vi "XCalib.vi"(7 "B [T]":dbl=1.0, 8 "error in (no error)":errorcluster, 10 "fileCalib":T1, 11 "DB calib":T10) -> (0 "error out":errorcluster, 2 "fileCalib out":T1, 3 "cam calib":T2={"incident ANGLE COMPENSATION"=[], "dp/B [MeV/C/B]"=[], "charge compensation"=[], "Momentum [MeV/C]"=[], "energyDependence Input"=[], "pixel angle (y)"=[], "dp [MeV/C/] "=[], "angle 2Dfor spectrumj"=[], "dp [MeV/C] 2D"=[], "charge compensation 2D"=[], "Screen&Camera 2"={"Screen Orientation"="Regular", "Screen angle"="Flat", "Lens"=enum."FL1-f8x08", "Calibration (mm/pix)"=1.0}, "ROI info"={"npix-X"=0, "npix-Y"=0, "Left [pix]"=0.0, "Top [pix]"=0.0}, "Y 2D full angle"=[], "calib pixel"={"y1(pixel)"=[], "y2(pixel)"=[], "dp/B [MeV/C/B] (pixel)"=[], "energyDependence Input(pixel)"=[], "bending angle [deg](pixel)"=[], "total path(pixel)"=[], "pixel angle (y)(pixel)"=[], "energy dependence (pixel)"=[], "charge compensation (pixel)"=[], "Momentum [MeV/C](pixel)"=[], "angular compensation(pixel)"=[]}, "2D"={"dp"=[], "chargeCompensation"=[], "angle"=[], "Momentum"=[]}, "UserROI"={"Width"=0.0, "Hight"=0.0, "OffsetX"=0.0, "OffsetY"=0.0}, "final"={"X"=[], "xi"=[], "delta momentum"=0.0, "Y"=[], "yi"=[], "angle (Y)"=[], "delta angle"=0.0, "scale delta angle"=0.0, "intraX"=0.0, "intraY"=0.0, "mask"=[]}, "B[T]"=0.0, "index"=0.0})   [LabVIEW 2013]
uses:
  calibPixel.ctl
  CamSettingSUB_TypDEf.ctl
  MagAnalysis_Online_Bella/SubVis/CamAndObj_TypDEf.ctl
  shared/OnOffTypeDef.ctl
  userROI.ctl
  shared/numericVariable_TypeDef.ctl
  CamRoiTypDef.ctl
  configTypDEf.ctl
  calib_Sub_Typdef.ctl
  ScreenCam2_TypDEf.ctl
  ROIInfo_TypDef.ctl
  2DTypDef.ctl
  finalCalibTypdef.ctl
  BaseDriver/BaseDriver.lvclass
panel:
  out "calib(pixel) out out 2":T6
  out "XY Graph":cluster{dbl[], "Array out":dbl[]}[](graph)
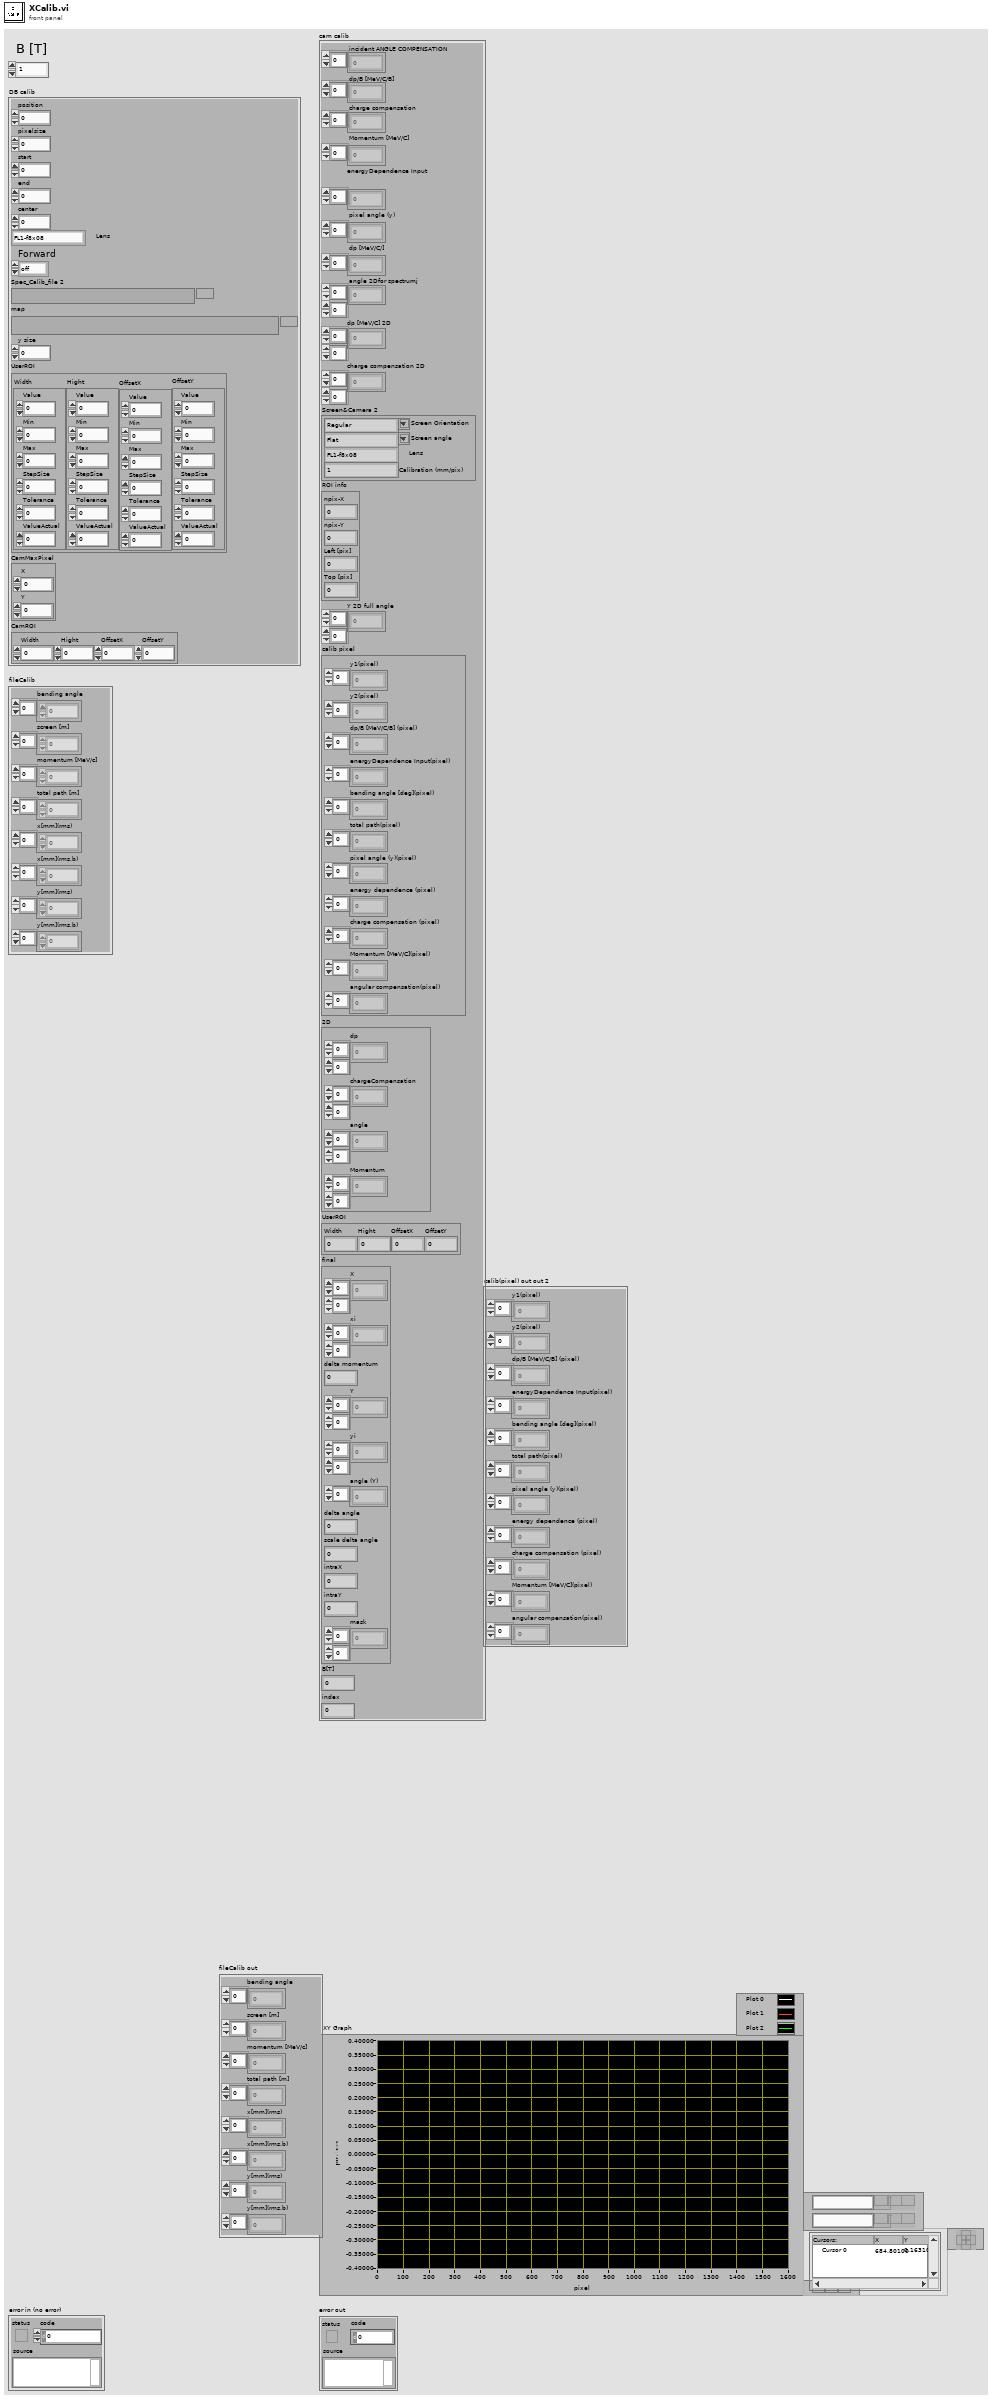
[diagram p1: front panel]
types:
  T1 = typedef "configTypDEf.ctl" = cluster{"bending angle":dbl[], "screen [m]":dbl[], "momentum [MeV/c]":dbl[], "total path [m]":dbl[], "x[mm](rms)":dbl[], "x[mm](rms,b)":dbl[], "y[mm](rms)":dbl[], "y[mm](rms,b)":dbl[]}
  T2 = typedef "calib_Sub_Typdef.ctl" = cluster{"incident ANGLE COMPENSATION":dbl[], "dp/B [MeV/C/B]":dbl[], "charge compensation":dbl[], "Momentum [MeV/C]":dbl[], "energyDependence Input":dbl[], "pixel angle (y)":dbl[], "dp [MeV/C/] ":dbl[], "angle 2Dfor spectrumj":dbl[][], "dp [MeV/C] 2D":dbl[][], "charge compensation 2D":dbl[][], "Screen&Camera 2":T3, "ROI info":T5, "Y 2D full angle":dbl[][], "calib pixel":T6, "2D":T7, "UserROI":T8, "final":T9, "B[T]":dbl, "index":dbl}
  T3 = typedef "ScreenCam2_TypDEf.ctl" = cluster{"Screen Orientation":string, "Screen angle":string, "Lens":T4, "Calibration (mm/pix)":dbl}
  T4 = typedef "CamAndObj_TypDEf.ctl" = enum16{"FL1-f8x08", "FL1-f8x06", "FL1-f8", "ch300-f50", "FL2G-f8", "FL3M14-f8", "FL3M14-f8x08", "FL3M14-f8x08(2x2)"}
  T5 = typedef "ROIInfo_TypDef.ctl" = cluster{"npix-X":i32, "npix-Y":i32, "Left [pix]":dbl, "Top [pix]":dbl}
  T6 = typedef "calibPixel.ctl" = cluster{"y1(pixel)":dbl[], "y2(pixel)":dbl[], "dp/B [MeV/C/B] (pixel)":dbl[], "energyDependence Input(pixel)":dbl[], "bending angle [deg](pixel)":dbl[], "total path(pixel)":dbl[], "pixel angle (y)(pixel)":dbl[], "energy dependence (pixel)":dbl[], "charge compensation (pixel)":dbl[], "Momentum [MeV/C](pixel)":dbl[], "angular compensation(pixel)":dbl[]}
  T7 = typedef "2DTypDef.ctl" = cluster{"dp":dbl[][], "chargeCompensation":dbl[][], "angle":dbl[][], "Momentum":dbl[][]}
  T8 = typedef "CamRoiTypDef.ctl" = cluster{"Width":dbl, "Hight":dbl, "OffsetX":dbl, "OffsetY":dbl}
  T9 = typedef "finalCalibTypdef.ctl" = cluster{"X":dbl[][], "xi":dbl[][], "delta momentum":dbl, "Y":dbl[][], "yi":dbl[][], "angle (Y)":dbl[], "delta angle":dbl, "scale delta angle":dbl, "intraX":dbl, "intraY":dbl, "mask":dbl[][]}
  T10 = typedef "CamSettingSUB_TypDEf.ctl" = cluster{"position":dbl, "pixelsize":dbl, "start":dbl, "end":dbl, "center":dbl, "Lens":T4, "Forward":T11, "Spec_Calib_file 2":path, "map":path, "y size":i32, "UserROI":T12, "CamMaxPixel":cluster{"X":i32, "Y":i32}, "CamROI":T8}
  T11 = typedef "OnOffTypeDef.ctl" = enum16{"off", "on"}
  T12 = typedef "userROI.ctl" = cluster{"Width":T13, "Hight":T13, "OffsetX":T13, "OffsetY":T13}
  T13 = typedef "BaseDriver.lvclass/numericVariable_TypeDef.ctl" = cluster{"Value":dbl, "Min":dbl, "Max":dbl, "StepSize":dbl, "Tolerance":dbl, "ValueActual":dbl}
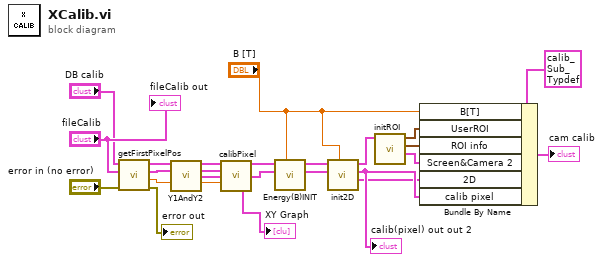
[diagram p0: block diagram]
diagram:
  n1 = call "getFirstPixelPos.vi"("error in (no error)"="error in (no error)", "Cluster"="fileCalib", "Cam 0"="DB calib") -> ("error out"=→"error out":errorcluster, "first Pixel position"=w9:dbl, "Cluster out"=w5:T1, "Cam out"=w19:T10)  [unwired: 5 in]
  n2 = call "Y1AndY2.vi"("Cam 0"=w19, "Cluster"=w5, "position"=w9) -> ("Cam 1"=w20:T10, "Clustero ut"=w10:T1, "calib(pixel)"=w11:T6, "position 2"=w12:dbl)  [unwired: 9 in]
  n3 = call "calibPixel.vi"("Cam 1"=w20, "Clustero ut"=w10, "calib(pixel) in"=w11, "first Pixel position"=w12) -> ("Cam out"=w21:T10, "calib(pixel) out"=w16:T6, "XY Graph"=→"XY Graph":cluster{dbl[], "Array out":dbl[]}[])  [unwired: 9 in]
  n4 = call "Energy(B)INIT.vi"("B [T] in"="B [T]", "calib(pixel) out in"=w16, "Cam in"=w21) -> ("calib(pixel) out out"=w17:T6, "Cam out 2"=w22:T10)  [unwired: 7 in]
  n5 = call "init2D.vi"("B [T]"="B [T]", "calib(pixel) out out"=w17, "Cam out"=w22) -> ("2D"=w18:T7, "calib(pixel) out out 2"=w25:T6, "Cam out 2"=w23:T10)  [unwired: 6 in]
  "calib(pixel) out out 2" <- w25
  n6 = call "initROI.vi"("Cam out"=w23) -> ("Screen&Camera 2"=w14:T3, "ROI info"=w4:T5, "UserROI"=w15:T8)  [unwired: 8 in]
  n7 = Bundle By Name(cluster=T2 {"incident ANGLE COMPENSATION"=[], "dp/B [MeV/C/B]"=[], "charge compensation"=[], "Momentum [MeV/C]"=[], "energyDependence Input"=[], "pixel angle (y)"=[], "dp [MeV/C/] "=[], "angle 2Dfor spectrumj"=[], "dp [MeV/C] 2D"=[], "charge compensation 2D"=[], "Screen&Camera 2"={"Screen Orientation"="", "Screen angle"="", "Lens"=enum."FL1-f8x08", "Calibration (mm/pix)"=0.0}, "ROI info"={"npix-X"=0, "npix-Y"=0, "Left [pix]"=0.0, "Top [pix]"=0.0}, "Y 2D full angle"=[], "calib pixel"={"y1(pixel)"=[], "y2(pixel)"=[], "dp/B [MeV/C/B] (pixel)"=[], "energyDependence Input(pixel)"=[], "bending angle [deg](pixel)"=[], "total path(pixel)"=[], "pixel angle (y)(pixel)"=[], "energy dependence (pixel)"=[], "charge compensation (pixel)"=[], "Momentum [MeV/C](pixel)"=[], "angular compensation(pixel)"=[]}, "2D"={"dp"=[], "chargeCompensation"=[], "angle"=[], "Momentum"=[]}, "UserROI"={"Width"=0.0, "Hight"=0.0, "OffsetX"=0.0, "OffsetY"=0.0}, "final"={"X"=[], "xi"=[], "delta momentum"=0.0, "Y"=[], "yi"=[], "angle (Y)"=[], "delta angle"=0.0, "scale delta angle"=0.0, "intraX"=0.0, "intraY"=0.0, "mask"=[]}, "B[T]"=0.0, "index"=0.0} ("cam calib"), "B[T]"="B [T]", "UserROI"=w15, "ROI info"=w4, "Screen&Camera 2"=w14, "2D"=w18, "calib pixel"=w25) -> (→"cam calib":T2)
  "fileCalib out" <- "fileCalib"
